vi "Reset Meas v 2.vi"(11 "simulate":bool) -> (1 "Error USB #2":bool, 2 "Error USB #1":bool, 3 "Error USB #0":bool)   [LabVIEW 2013]
panel:
  out "Message":string
  in  "End Reset Routine":bool
  # "RESET BUSY"
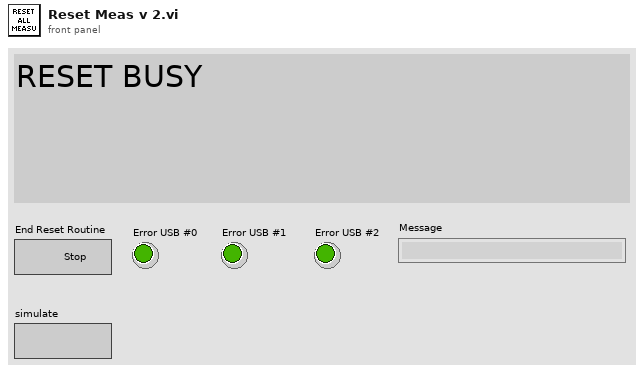
[diagram p1: front panel]
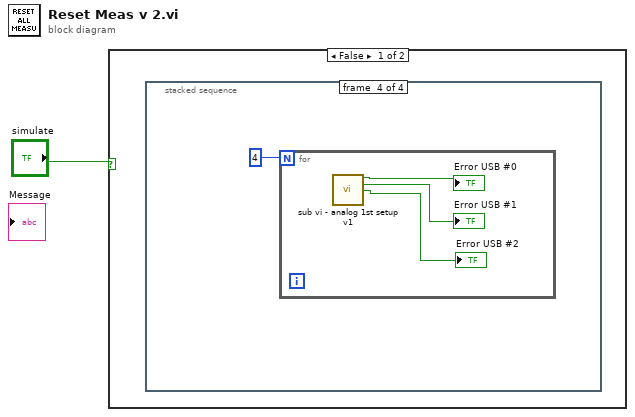
[diagram p0: block diagram]
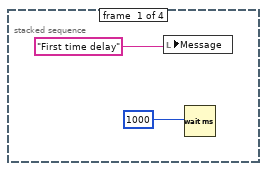
[diagram p2: hidden frame]
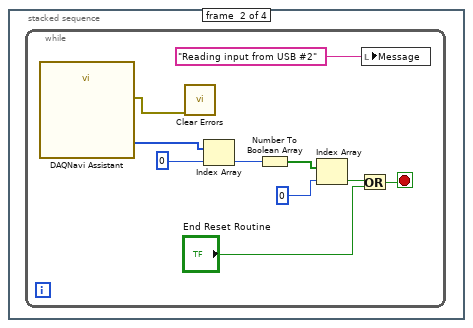
[diagram p3: hidden frame]
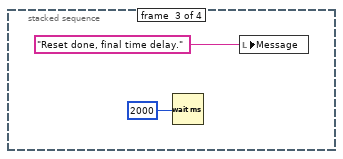
[diagram p4: hidden frame]
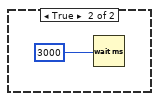
[diagram p5: hidden frame]
diagram:
  n1 = case shown="False" "simulate" {
    frame False {
      n2 = stacked-sequence {
        frame #0 {
          n3 = local write "Message"("First time delay") -> ()
          n4 = Wait (ms)(milliseconds to wait=1000) -> ()  [unwired: 1 out]
        }
        frame #1 {
          n5 = while {
            stop <- w8 stop-if-true
            n6 = call "DAQNavi Assistant"() -> ("error out"=w5:errorcluster, "dataOut(U8Array)"=w9:u8[])  [unwired: 26 in]
            n7 = call <vilib>:"Clear Errors.vi"("error in (no error)"=w5) -> ()  [unwired: 6 in, 1 out]
            n8 = Index Array(array=w9, index=0) -> (element=w11:u8)
            n9 = Number To Boolean Array(number=w11) -> (Boolean array=w12:bool[])
            n10 = Index Array(array=w12, index=0) -> (element=w7:bool)
            n11 = Or(x=w7, y="End Reset Routine") -> (x .or. y?=w8:bool)
            n12 = local write "Message"("Reading input from USB #2") -> ()
          }
        }
        frame #2 {
          n13 = Wait (ms)(milliseconds to wait=2000) -> ()  [unwired: 1 out]
          n14 = local write "Message"("Reset done, final time delay.") -> ()
        }
        frame #3 {
          n15 = for {
            N: 4 -> [_]
            n16 = call "sub vi - analog 1st setup v1.vi"() -> ("Error USB #0"=→"Error USB #0":bool, "Error USB #1"=→"Error USB #1":bool, "Error USB #2"=→"Error USB #2":bool)  [unwired: 9 in, 4 out]
          }
        }
      }
    }
    frame True {
      n17 = Wait (ms)(milliseconds to wait=3000) -> ()  [unwired: 1 out]
    }
  }
